vi "Define_Matrices_sub.vi"(11 "Sampling Freqauency (Hz)":dbl=10000.0) -> (1 "Q = GQG'":T1, 2 "G Matrix":T1, 3 "H Matrix":T1=[[0.0, 1.0], [9.81, 0.0]], 4 "F  Matrix":T1=[[1.0, 0.0001], [0.0, 1.0]], 5 "R Matrix":T1=[[1e-10, 0.0], [0.0, 1e-11]])   [LabVIEW 2020]
uses:
  <vilib>/Analysis/Matrix/Datatypes/RealMatrix.ctl
  <vilib>/Analysis/baseanly.llb/Real A x B.vi
  <vilib>/Analysis/Matrix/Numeric/Conversions/Array To Matrix - RA2.vi
  <vilib>/Analysis/7linalg.llb/Real Transpose Matrix.vi
  <vilib>/Analysis/Matrix/NI_Matrix.lvlib
  <vilib>/Analysis/NI_AALBase.lvlib
  <vilib>/Analysis/NI_AALPro.lvlib
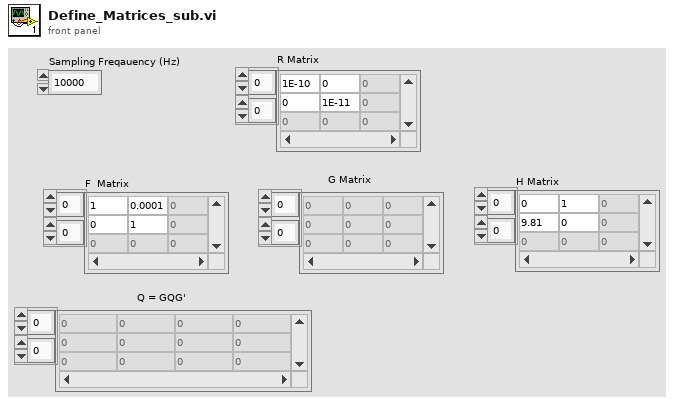
[diagram p1: front panel]
types:
  T1 = typedef "NI_Matrix.lvlib/RealMatrix.ctl" = dbl[][]
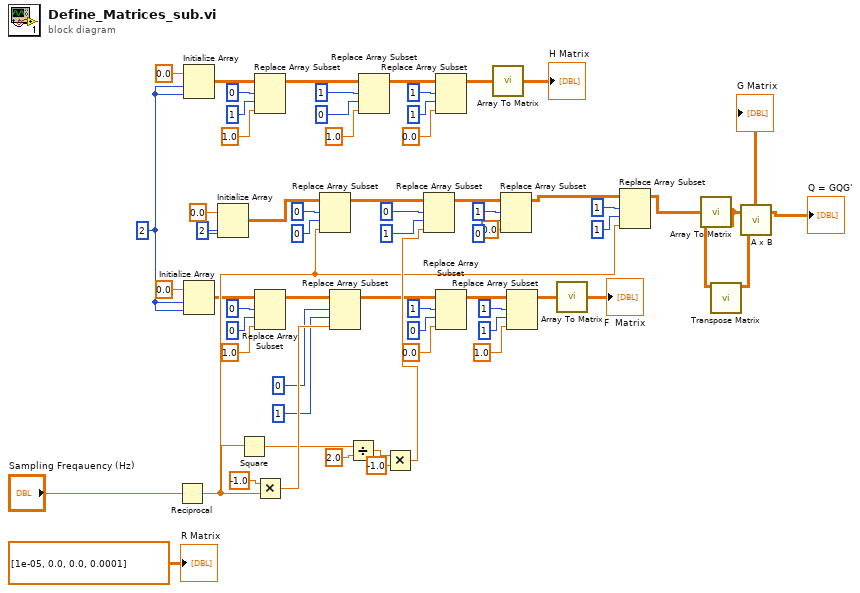
[diagram p0: block diagram]
diagram:
  w41 = 2 ("dimension size")
  w39 = 2 ("dimension size")
  n1 = Reciprocal(x="Sampling Freqauency (Hz)") -> (1/x=w56:dbl)
  n2 = Initialize Array(0.0 ("element"), w39, w39) -> (w13:dbl[][])
  n3 = Initialize Array(0.0 ("element"), w39, w39) -> (w34:dbl[][])
  n4 = Initialize Array(0.0 ("element"), w41, w41) -> (w50:dbl[][])
  n5 = Square(x=w56) -> (x^2=w19:dbl)
  n6 = Replace Array Subset(array=w13, new element=1.0 ("new element/subarray"), index (row)=0, index (col)=1 ("disabled index (col)")) -> (w9:dbl[][])
  n7 = Replace Array Subset(array=w34, new element=1.0 ("new element/subarray"), index (row)=0, index (col)=0 ("disabled index (col)")) -> (w30:dbl[][])
  n8 = Multiply(x=-1.0, y=w56) -> (x*y=w54:dbl)
  n9 = Replace Array Subset(array=w50, new element=w56, index (row)=0, index (col)=0 ("disabled index (col)")) -> (w46:dbl[][])
  n10 = Replace Array Subset(array=w30, new element=w54, index (row)=0, index (col)=1 ("disabled index (col)")) -> (w27:dbl[][])
  n11 = Divide(x=w19, y=2.0) -> (x/y=w58:dbl)
  n12 = Replace Array Subset(array=w9, new element=1.0 ("new element/subarray"), index (row)=1, index (col)=0 ("disabled index (col)")) -> (w5:dbl[][])
  n13 = Multiply(x=w58, y=-1.0) -> (x*y=w60:dbl)
  n14 = Replace Array Subset(array=w46, new element=w60, index (row)=0, index (col)=1 ("disabled index (col)")) -> (w49:dbl[][])
  n15 = Replace Array Subset(array=w5, new element=0.0 ("new element/subarray"), index (row)=1, index (col)=1 ("disabled index (col)")) -> (w2:dbl[][])
  n16 = Replace Array Subset(array=w27, new element=0.0 ("new element/subarray"), index (row)=1, index (col)=0 ("disabled index (col)")) -> (w23:dbl[][])
  n17 = call-poly <vilib>:"Array To Matrix.vi"("Real 2D Array"=w2) -> ("Real Matrix"=→"H Matrix":T1)
  n18 = Replace Array Subset(array=w49, new element=0.0 ("new element/subarray"), index (row)=1, index (col)=0 ("disabled index (col)")) -> (w53:dbl[][])
  n19 = Replace Array Subset(array=w23, new element=1.0 ("new element/subarray"), index (row)=1, index (col)=1 ("disabled index (col)")) -> (w4:dbl[][])
  n20 = call-poly <vilib>:"Array To Matrix.vi"("Real 2D Array"=w4) -> ("Real Matrix"=→"F  Matrix":T1)
  n21 = Replace Array Subset(array=w53, new element=w56, index (row)=1, index (col)=1 ("disabled index (col)")) -> (w57:dbl[][])
  n22 = call-poly <vilib>:"Array To Matrix.vi"("Real 2D Array"=w57) -> ("Real Matrix"=w62:T1)
  "G Matrix" <- w62
  n23 = call-poly <vilib>:"Transpose Matrix.vi"("Input Matrix"=w62) -> ("Matrix Transpose"=w63:T1)  [unwired: 9 in, 1 out]
  n24 = call-poly <vilib>:"A x B.vi"("B"=w63, "A"=w62) -> ("A x B"=→"Q = GQG'":T1)  [unwired: 1 out]
  "R Matrix" <- T1 [[1e-05, 0.0], [0.0, 0.0001]] ("F  Matrix")
